vi "Control Digital Input - Static.vi"(8 "error in":errorcluster, 11 "Line(s)":tag="Dev1/port0/line0:7") -> (0 "error out":errorcluster, 2 "Hexadecimal Data":u32 format="%x", 3 "Boolean Data":bool[](array[boolean]))   [LabVIEW 2016]
doc: "This example demonstrates how to acquire the state of digital lines based off of software timing.\n\nFor instructions on how to connect your signals to the DAQ device, refer to your device documentation."
uses:
  <vilib>/DAQmx/read.llb/DAQmx Read (Digital 1D Bool 1Chan 1Samp).vi
  <vilib>/DAQmx/create/channels.llb/DAQmx Create Channel (DI-Digital Input).vi
  <vilib>/DAQmx/miscellaneous.llb/DAQmx Fill In Error Info.vi
panel:
  # "Channel Settings"
  # "Acquired Data"
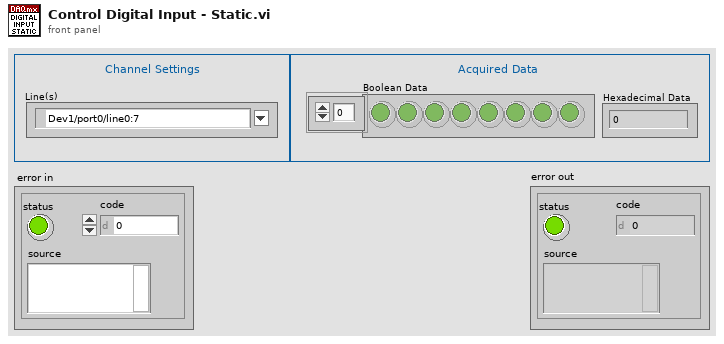
[diagram p1: front panel]
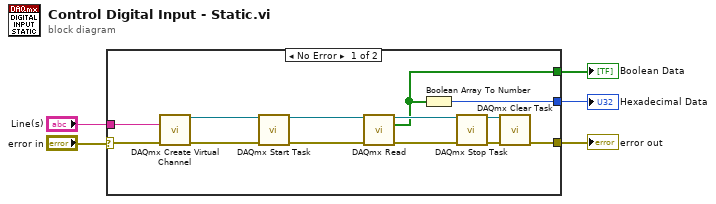
[diagram p0: block diagram]
diagram:
  n1 = case shown="No Error" "error in" {
    selector: "error in" -> [w6 w19]
    tunnel: "Line(s)" -> [w16 _]
    tunnel: [w9 _] -> w4
    tunnel: [w8 _] -> w3
    tunnel: [w7 w19] -> w2
    frame No Error {
      n2 = call-poly <vilib>:"DAQmx Create Virtual Channel.vi"("lines"=w16, "error in"=w6) -> ("task out"=w14:refnum<k21>, "error out"=w15:errorcluster)  [unwired: 12 in]
      n3 = call <vilib>:"DAQmx Start Task.vi"("task/channels in"=w14, "error in"=w15) -> ("task out"=w18:refnum<k21>, "error out"=w17:errorcluster)  [unwired: 12 in]
      n4 = call-poly <vilib>:"DAQmx Read.vi"("task/channels in"=w18, "error in"=w17) -> ("task out"=w13:refnum<k21>, "data"=w9:bool[], "error out"=w12:errorcluster)  [unwired: 11 in]
      n5 = Boolean Array To Number(Boolean array=w9) -> (number=w8:u32)
      n6 = call <vilib>:"DAQmx Stop Task.vi"("task/channels in"=w13, "error in"=w12) -> ("task out"=w11:refnum<k21>, "error out"=w10:errorcluster)  [unwired: 12 in]
      n7 = call <vilib>:"DAQmx Clear Task.vi"("task in"=w11, "error in"=w10) -> ("error out"=w7:errorcluster)  [unwired: 13 in]
    }
    frame Error {
    }
  }
  "Boolean Data" <- w4
  "Hexadecimal Data" <- w3
  "error out" <- w2
